vi "SetFrequencySpan.vi"(8 "error in (no error)":errorcluster, 9 "Frequency Span[Hz]":dbl, 10 "Analyzer (0: A0)":i32(ring) items=["A0", "A1"], 11 "VISA resource name":refnum<visa-resource-name>) -> (0 "error out":errorcluster, 3 "VISA resource name out":refnum<visa-resource-name>)   [LabVIEW 2014, in "Stanford Research SR1.lvlib"]
doc: "Sets the actual bandwidth."
uses:
  Stanford Research SR1.lvlib
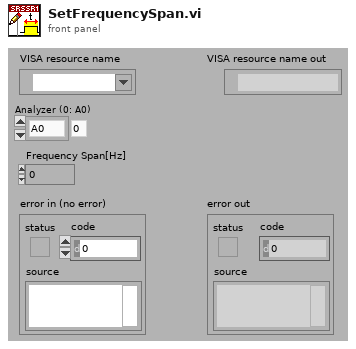
[diagram p1: front panel]
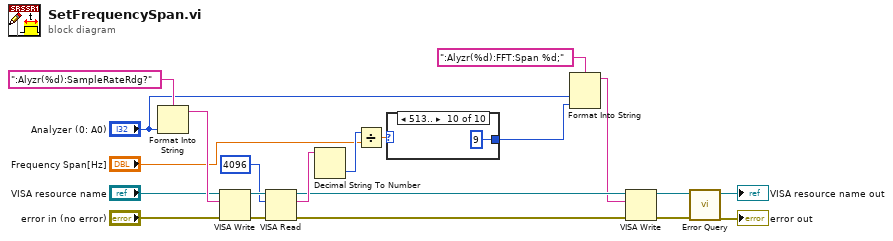
[diagram p0: block diagram]
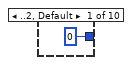
[diagram p2: hidden frame]
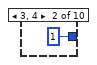
[diagram p3: hidden frame]
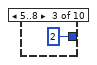
[diagram p4: hidden frame]
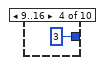
[diagram p5: hidden frame]
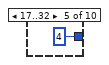
[diagram p6: hidden frame]
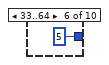
[diagram p7: hidden frame]
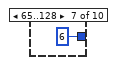
[diagram p8: hidden frame]
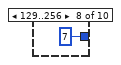
[diagram p9: hidden frame]
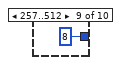
[diagram p10: hidden frame]
diagram:
  n1 = Format Into String(format string=":Alyzr(%d):SampleRateRdg?", "Analyzer (0: A0)") -> (resulting string=w15:string)  [unwired: 2 in, 1 out]
  n2 = VISA Write(VISA resource name="VISA resource name", write buffer=w15, error in (no error)="error in (no error)") -> (VISA resource name out=w16:refnum<visa-resource-name>, error out=w17:errorcluster)  [unwired: 1 out]
  n3 = VISA Read(VISA resource name=w16, byte count=4096, error in (no error)=w17) -> (VISA resource name out=w9:refnum<visa-resource-name>, read buffer=w13:string, error out=w10:errorcluster)  [unwired: 1 out]
  n4 = Decimal String To Number(string=w13) -> (number=w6:i32)  [unwired: 2 in, 1 out]
  n5 = Divide(x=w6, y="Frequency Span[Hz]") -> (x/y=w4:dbl)
  n6 = case shown="513.." w4 {
    tunnel: [0 1 2 3 4 5 6 7 8 9] -> w1
    frame ..2, Default {
    }
    frame 3, 4 {
    }
    frame 5..8 {
    }
    frame 9..16 {
    }
    frame 17..32 {
    }
    frame 33..64 {
    }
    frame 65..128 {
    }
    frame 129..256 {
    }
    frame 257..512 {
    }
    frame 513.. {
    }
  }
  n7 = Format Into String(format string=":Alyzr(%d):FFT:Span %d;", "Analyzer (0: A0)", w1) -> (resulting string=w3:string)  [unwired: 2 in, 1 out]
  n8 = VISA Write(VISA resource name=w9, write buffer=w3, error in (no error)=w10) -> (VISA resource name out=w8:refnum<visa-resource-name>, error out=w7:errorcluster)  [unwired: 1 out]
  n9 = call "Error Query.vi"("error in (no error)"=w7, "VISA resource name"=w8) -> ("error out"=→"error out":errorcluster, "VISA resource name out"=→"VISA resource name out":refnum<visa-resource-name>)  [unwired: 6 in, 2 out]
